vi "BRig_dataLC_ENL2_First_Prob_l1.vi"() -> (2 "output_ENL2_First_Prob":i32)   [LabVIEW 2014]
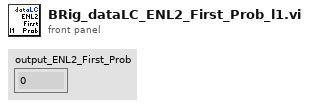
[diagram p1: front panel]
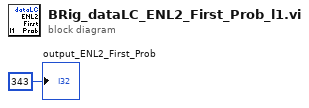
[diagram p0: block diagram]
diagram:
  "output_ENL2_First_Prob" <- 343 ("output_iBlock")
